vi "Write Device Resource.vi"(8 "error in (no error)":errorcluster, 10 "Device Resource":refnum<visa-resource-name>, 11 "DG645 in":refnum<class "DG645.lvclass">) -> (0 "error out":errorcluster, 3 "DG645 out":refnum<class "DG645.lvclass">)   [LabVIEW 2018, in "DG645.lvlib" / "DG645.lvclass"]
uses:
  DG645.lvclass
  DG645.lvclass/DG645.ctl
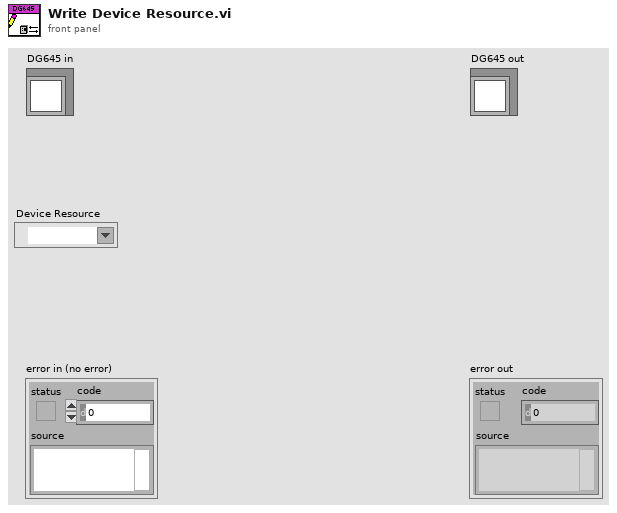
[diagram p1: front panel]
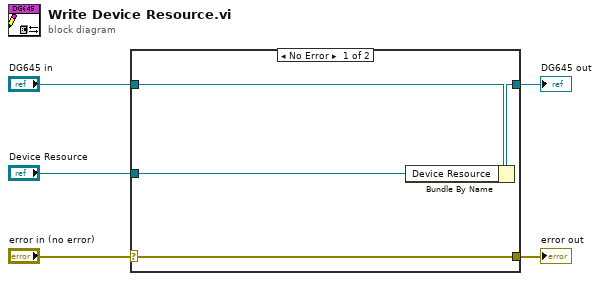
[diagram p0: block diagram]
diagram:
  n1 = case shown="No Error" "error in (no error)" {
    selector: "error in (no error)" -> [w9 w10]
    tunnel: [w9 w10] -> w4
    tunnel: [w7 w11] -> w2
    tunnel: "DG645 in" -> [w8 w11]
    tunnel: "Device Resource" -> [w6 _]
    frame No Error {
      n2 = Bundle By Name(cluster=w8, "Device Resource"=w6) -> (w7:refnum<class "DG645.lvclass">)
    }
    frame Error {
    }
  }
  "error out" <- w4
  "DG645 out" <- w2
